vi "From SpecificCluste To SettingsCluster.vi"(7 "variant (destination)":variant, 8 "error in (no error)":errorcluster, 9 "Seperator (\"\")":string="Channel 1", 11 "variant  (source)":variant) -> (0 "error  out":errorcluster, 1 "Seperator out":string="Channel 1", 3 "variant out":variant)   [LabVIEW 2011]
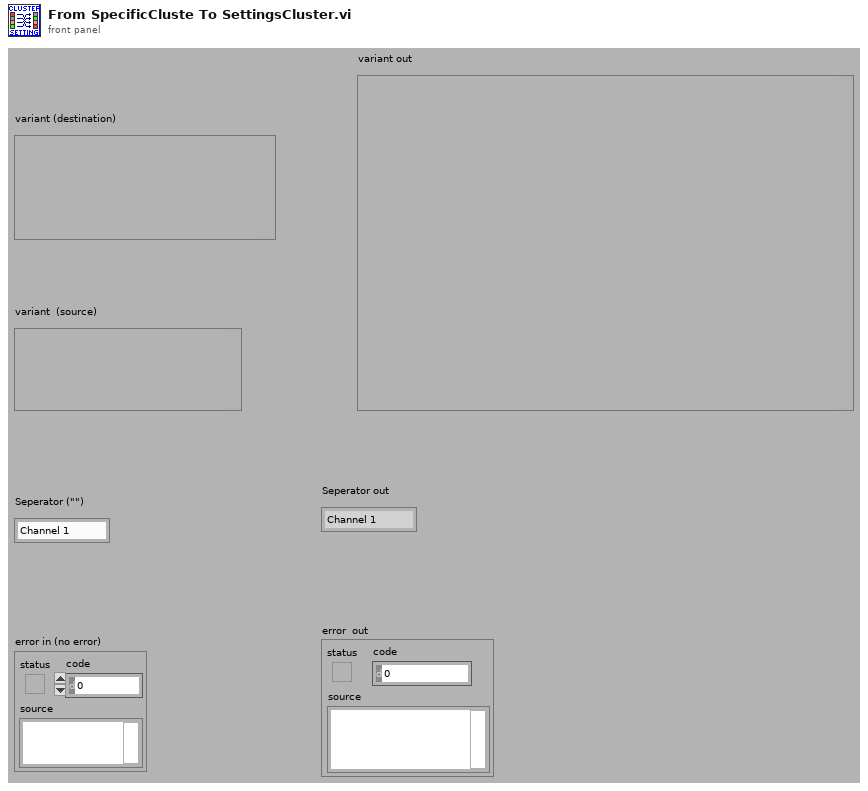
[diagram p1: front panel]
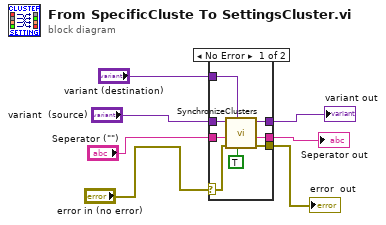
[diagram p0: block diagram]
diagram:
  n1 = case shown="No Error" "error in (no error)" {
    selector: "error in (no error)" -> [w8 w18]
    tunnel: "variant  (source)" -> [w14 _]
    tunnel: "Seperator (\"\")" -> [w13 w17]
    tunnel: [w12 w18] -> w5
    tunnel: [w11 w17] -> w4
    tunnel: [w10 w16] -> w3
    tunnel: "variant (destination)" -> [w9 w16]
    frame No Error {
      n2 = call "SynchronizeClusters.vi"("toSettings"=TRUE, "variant (destination)"=w9, "error in (no error)"=w8, "Seperator (\"\")"=w13, "variant  (source)"=w14) -> ("error  out"=w12:errorcluster, "Seperator out"=w11:string, "variant out"=w10:variant)  [unwired: 4 in]
    }
    frame Error {
    }
  }
  "error  out" <- w5
  "Seperator out" <- w4
  "variant out" <- w3
